vi "Read pathOfSalMonitor.vi"(8 "error in (no error)":errorcluster, 11 "LibReader in":refnum<class "LibReader.lvclass">) -> (0 "error out":errorcluster, 2 "pathOfSalMonitor":path, 3 "LibReader out":refnum<class "LibReader.lvclass">)   [LabVIEW 2018, in "LibReader.lvclass"]
doc: "Read the path of SAL monitor."
uses:
  LibReader.lvclass
  LibReader.lvclass/LibReader.ctl
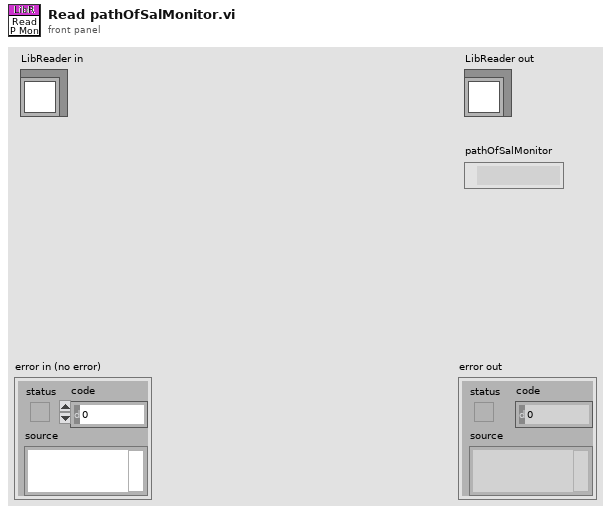
[diagram p1: front panel]
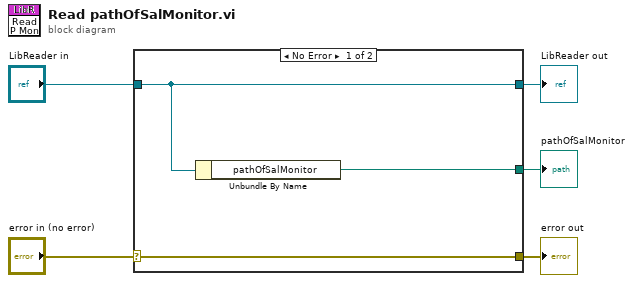
[diagram p0: block diagram]
diagram:
  n1 = case shown="No Error" "error in (no error)" {
    selector: "error in (no error)" -> [w8 w9]
    tunnel: [w8 w9] -> w4
    tunnel: [w7 w10] -> w2
    tunnel: "LibReader in" -> [w7 w10]
    tunnel: [w6 _] -> w1
    frame No Error {
      n2 = Unbundle By Name(w7) -> ("pathOfSalMonitor"=w6:path)
    }
    frame Error {
    }
  }
  "error out" <- w4
  "LibReader out" <- w2
  "pathOfSalMonitor" <- w1
